vi "Frequency Word to Frequency .vi"(9 "DDS clock":dbl=125000000.0 format="%_17p", 10 "DDS modulus":i64=15120 format="0x%x (%d)", 11 "Frequency word":i64=15120 format="0x%x (%d)") -> (3 "Frequency":dbl format="%_19p")   [LabVIEW 2019]
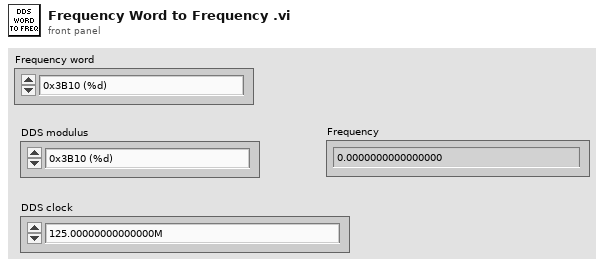
[diagram p1: front panel]
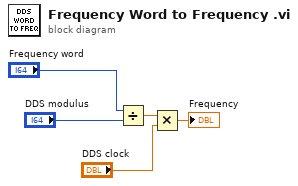
[diagram p0: block diagram]
diagram:
  n1 = Divide(x="Frequency word", y="DDS modulus") -> (x/y=w5:dbl)
  n2 = Multiply(x=w5, y="DDS clock") -> (x*y=→"Frequency":dbl)
